vi "Read_Code_Liniarity.vi"(2 "Repeat":i32=1 min=1 max=100, 5 "Port_No":u16=1444, 7 "Core_No":u16=1, 9 "ADC_Controls":T2={"ACQPS"=8, "Break_PT"=0, "Ref_Mod_Sel"=enum."Int_Ref_2P5", "Ref_Sel(Int/Ext)"=enum."Ext", "ADC"=enum."C", "Channel"=15, "LV_samples"=8194, "AGPIO_SEL"=0.0, "LV_perscale"=2, "ODIV"=1, "IMULT"=12}, 11 "error in":errorcluster) -> (4 "max value":u32=4056, 6 "AvgCode":dbl=2038.3436279296875, 8 "min value":u32=20, 15 "error out":errorcluster)   [LabVIEW 2019]
uses:
  Ctrls/ADC_CTRL.ctl
  <userlib>/_TI-LA/Reusable/CCS/APIs/CCS.lvlib
  <userlib>/_TI-LA/Reusable/CCS/APIs/Data/Polymorphics/Read Data From Address - U16 Array.vi
panel:
  in  "Refrence":dbl=2.5 format="%#_13g"
  in  "Sine_Wave_Data_file (use dialog)":path=path "D:/Projects/C2000/Grande/Data/ADC/Group_2/ID_406_AC_Specs/New Text Document.txt"
  out "Tot-Error":u32=4036
  out "Voltage":dbl=1.2441062182188034
  out "ADC_No":u16=2
  out "Waveform Graph":u32[](graph)
  out "Read Data[]":u32[](array[numeric]) format="%#.0f"
  # "1P65-0/2P5-1_Mode_Sel"
  # "LV_Break  = 0;\nUint16 LV_Repeat = 0;\nUint16 LV_Config = 0;\nUint16 LV_samples = 8192;\nUint16 LV_prescale = 2;\nUint16 LV_acqps = 25;\nUint16 LV_AGPIO_TEST = 0;\nUint32 LV_Avg = 0;\nUint16 LV_adcref=   1; // Internal Reference = 0\nUint16 LV_int2p5en= 1; // 2.5V Reference select = 1\nUint16 LV_adcmod =  2; // Adc sel A-0,B-1 & C-2\nUint16 LV_adcchan = 0; // Selecting ADC Channel\nUint16 LV_SYS_MULT =10;"
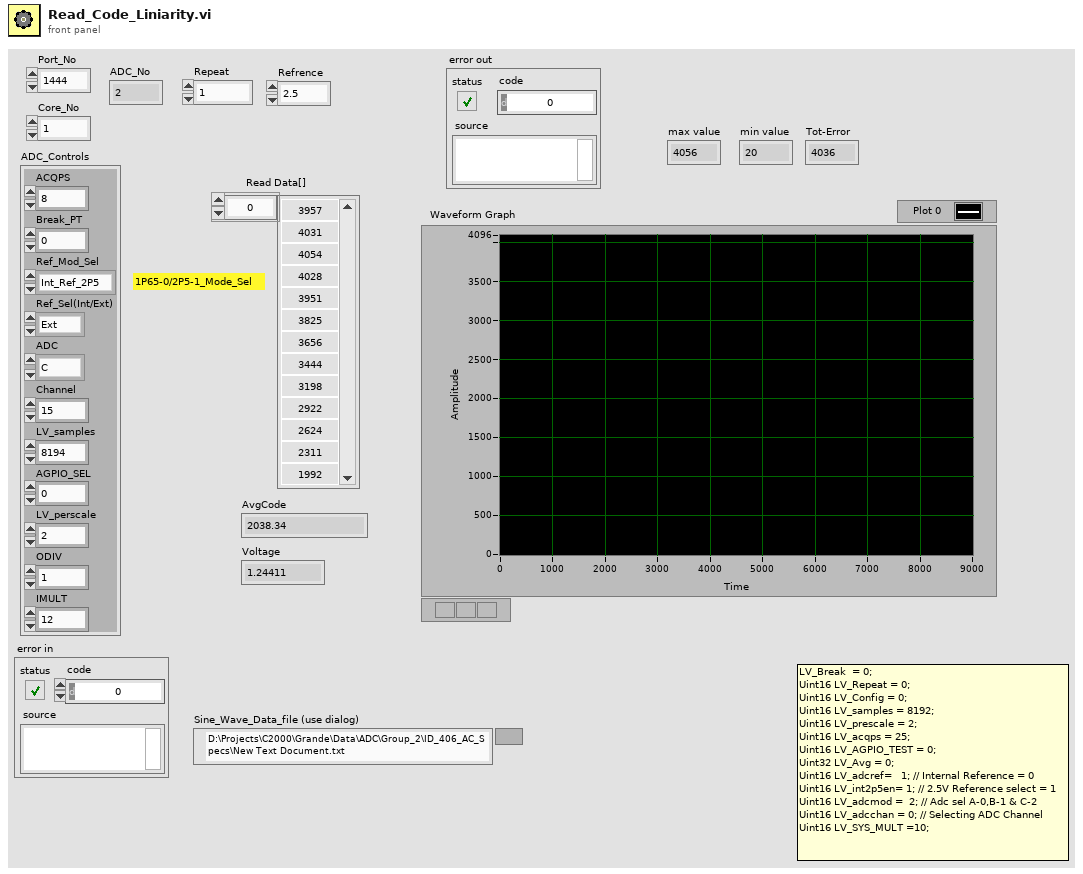
[diagram p1: front panel]
types:
  T1 = typedef "ADC_CTRL.ctl" = enum16{"A", "B", "C"}
  T2 = cluster{"ACQPS":u16, "Break_PT":u16, "Ref_Mod_Sel":enum16{"Int_Ref_1P65", "Int_Ref_2P5"}, "Ref_Sel(Int/Ext)":enum16{"Int", "Ext"}, "ADC":T1, "Channel":u16, "LV_samples":u16, "AGPIO_SEL":dbl, "LV_perscale":u16, "ODIV":u16, "IMULT":u16}
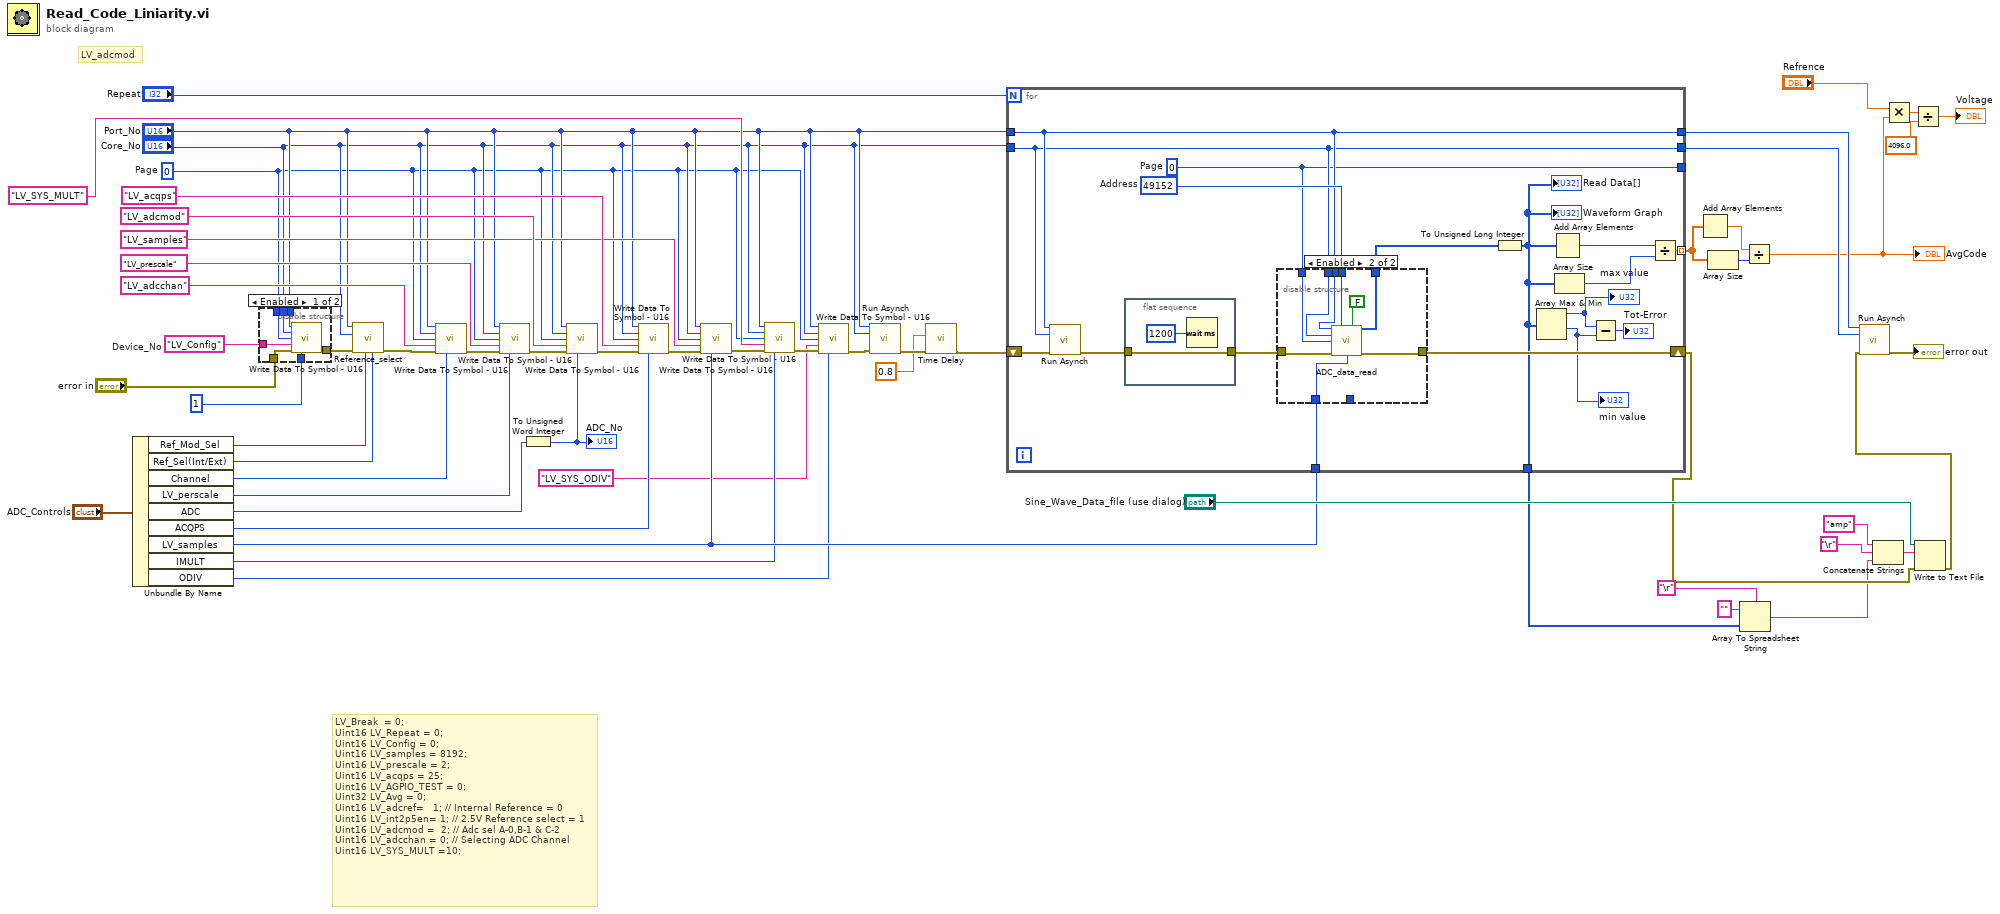
[diagram p0: block diagram]
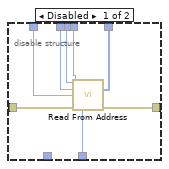
[diagram p3: hidden frame]
diagram:
  w40 = "LV_Config"  # Device_No
  w4 = 0  # Page
  # "LV_Break  = 0;\nUint16 LV_Repeat = 0;\nUint16 LV_Config = 0;\nUint16 LV_samples = 8192;\nUint16 LV_prescale = 2;\nUint16 LV_acqps = 25;\nUint16 LV_AGPIO_TEST = 0;\nUint32 LV_Avg = 0;\nUint16 LV_adcref=   1; // Internal Reference = 0\nUint16 LV_int2p5en= 1; // 2.5V Reference select = 1\nUint16 LV_adcmod =  2; // Adc sel A-0,B-1 & C-2\nUint16 LV_adcchan = 0; // Selecting ADC Channel\nUint16 LV_SYS_MULT =10;"
  # "LV_adcmod"
  n1 = Unbundle By Name("ADC_Controls") -> ("Ref_Mod_Sel"=w31:enum16{"Int_Ref_1P65", "Int_Ref_2P5"}, "Ref_Sel(Int/Ext)"=w30:enum16{"Int", "Ext"}, "Channel"=w29:u16, "LV_perscale"=w28:u16, "ADC"=w27:T1, "ACQPS"=w26:u16, "LV_samples"=w9:u16, "IMULT"=w2:u16, "ODIV"=w3:u16)
  n2 = disable-structure shown="Enabled" {
    disable-tunnel: "error in" -> [w65 _]
    disable-tunnel: w40 -> [w64 _]
    disable-tunnel: w4 -> [w63 _]
    disable-tunnel: [w62 _] -> w39
    disable-tunnel: u16 1 ("Write Data") -> [w61 _]
    disable-tunnel: "Port_No" -> [w60 _]
    disable-tunnel: "Core_No" -> [w59 _]
    frame Enabled {
      n3 = call <userlib>:"Write Data To Symbol - U16.vi"("Port Number"=w60, "Core Number"=w59, "Page"=w63, "Symbol Name"=w64, "error in"=w65, "Write Data"=w61) -> ("error out"=w62:errorcluster)  [unwired: 7 in, 2 out]
    }
    frame Disabled {
    }
  }
  n4 = call "Reference_select.vi"("Ref_Sel(Int/Ext)"=w30, "INT_Ref_Sel"=w31, "error in"=w39, "Core Number"="Core_No", "Port Number"="Port_No") -> ("error out"=w38:errorcluster)  [unwired: 6 in]
  n5 = call <userlib>:"Write Data To Symbol - U16.vi"("Port Number"="Port_No", "Core Number"="Core_No", "Page"=w4, "Symbol Name"="LV_adcchan", "error in"=w38, "Write Data"=w29) -> ("error out"=w57:errorcluster)  [unwired: 7 in, 2 out]
  n6 = call <userlib>:"Write Data To Symbol - U16.vi"("Port Number"="Port_No", "Core Number"="Core_No", "Page"=w4, "Symbol Name"="LV_prescale", "error in"=w57, "Write Data"=w28) -> ("error out"=w56:errorcluster)  [unwired: 7 in, 2 out]
  n7 = To Unsigned Word Integer(number=w27) -> (unsigned 16bit integer=w47:u16)
  "ADC_No" <- w47
  n8 = call <userlib>:"Write Data To Symbol - U16.vi"("Port Number"="Port_No", "Core Number"="Core_No", "Page"=w4, "Symbol Name"="LV_adcmod", "error in"=w56, "Write Data"=w47) -> ("error out"=w58:errorcluster)  [unwired: 7 in, 2 out]
  n9 = call <userlib>:"Write Data To Symbol - U16.vi"("Port Number"="Port_No", "Core Number"="Core_No", "Page"=w4, "Symbol Name"="LV_acqps", "error in"=w58, "Write Data"=w26) -> ("error out"=w51:errorcluster)  [unwired: 7 in, 2 out]
  n10 = call <userlib>:"Write Data To Symbol - U16.vi"("Port Number"="Port_No", "Core Number"="Core_No", "Page"=w4, "Symbol Name"="LV_samples", "error in"=w51, "Write Data"=w9) -> ("error out"=w11:errorcluster)  [unwired: 7 in, 2 out]
  n11 = call <userlib>:"Write Data To Symbol - U16.vi"("Port Number"="Port_No", "Core Number"="Core_No", "Page"=w4, "Symbol Name"="LV_SYS_MULT", "error in"=w11, "Write Data"=w2) -> ("error out"=w8:errorcluster)  [unwired: 7 in, 2 out]
  n12 = call <userlib>:"Write Data To Symbol - U16.vi"("Port Number"="Port_No", "Core Number"="Core_No", "Page"=w4, "Symbol Name"="LV_SYS_ODIV", "error in"=w8, "Write Data"=w3) -> ("error out"=w7:errorcluster)  [unwired: 7 in, 2 out]
  n13 = call <userlib>:"Run Asynch.vi"("Port Number"="Port_No", "Core Number"="Core_No", "error in"=w7) -> ("error out"=w25:errorcluster)  [unwired: 10 in, 2 out]
  n14 = call "Time Delay"("error in (no error)"=w25, "Delay Time (s)"=0.8) -> ("error out"=w24:errorcluster)  [unwired: 9 in]
  n15 = for {
    N: "Repeat" -> [_]
    tunnel: [w79] -> w54 mode=indexing
    tunnel: "Port_No" -> [w75]
    tunnel: "Core_No" -> [w74]
    shift-right: [w78] -> w21
    shift-left: w24 -> [w77]
    tunnel: [w75] -> w50
    tunnel: [w74] -> w49
    tunnel: [w73] -> _
    tunnel: w9 -> [w67]
    tunnel: [w66] -> w13
    w81 = u32 49152  # Address
    w73 = 0  # Page
    n16 = call <userlib>:"Run Asynch.vi"("Port Number"=w75, "Core Number"=w74, "error in"=w77) -> ("error out"=w82:errorcluster)  [unwired: 10 in, 2 out]
    n17 = flat-sequence {
      tunnel: w82 -> [w100]
      tunnel: [w100] -> w72
      frame #0 {
        n18 = Wait (ms)(milliseconds to wait=u32 1200) -> ()  [unwired: 1 out]
      }
    }
    n19 = disable-structure shown="Enabled" {
      disable-tunnel: w81 -> [w90 w95]
      disable-tunnel: [w89 w97] -> w68
      disable-tunnel: [w88 w98] -> w78
      disable-tunnel: w75 -> [w87 w92]
      disable-tunnel: w74 -> [w86 w93]
      disable-tunnel: w73 -> [w85 w94]
      disable-tunnel: w72 -> [w84 w99]
      disable-tunnel: _ -> [w83 _]
      disable-tunnel: w67 -> [_ w96]
      frame Disabled {
        n20 = call-poly <userlib>:"Read From Address.vi"("Port Number"=w87, "Core Number"=w86, "Page"=w85, "Address"=w90, "error in"=w84, "Data Length"=w83) -> ("Read Data[]"=w89:u16[], "error out"=w88:errorcluster)  [unwired: 6 in, 2 out]
      }
      frame Enabled {
        n21 = call "ADC_data_read.vi"("Port Number"=w92, "Address"=w95, "Read_AVG ?"=FALSE, "Core Number"=w93, "Page"=w94, "error in (no error)"=w99, "Lv_Samples"=w96) -> ("Read Data[]"=w97:u16[], "error out"=w98:errorcluster)  [unwired: 6 in, 1 out]
      }
    }
    n22 = To Unsigned Long Integer(number=w68) -> (unsigned 32bit integer=w66:u32[])
    "Waveform Graph" <- w66
    "Read Data[]" <- w66
    n23 = Array Max & Min(array=w66) -> (max value=w71:u32, min value=w70:u32)  [unwired: 2 out]
    "max value" <- w71
    "min value" <- w70
    n24 = Add Array Elements(numeric array=w66) -> (sum=w80:u32)
    n25 = Array Size(array=w66) -> (size(s)=w76:i32)
    n26 = Subtract(x=w71, y=w70) -> (x-y=→"Tot-Error":u32)
    n27 = Divide(x=w80, y=w76) -> (x/y=w79:dbl)
  }
  n28 = Add Array Elements(numeric array=w54) -> (sum=w52:dbl)
  n29 = Array Size(array=w54) -> (size(s)=w53:i32)
  n30 = Array To Spreadsheet String(delimiter (Tab)="\r", array=w13, 3:"" ("format string")) -> (spreadsheet string=w14:string)
  n31 = Divide(x=w52, y=w53) -> (x/y=w46:dbl)
  "AvgCode" <- w46
  n32 = Concatenate Strings("amp", "\r", w14) -> (w18:string)
  n33 = Multiply(x="Refrence", y=w46) -> (x*y=w44:dbl)
  n34 = Divide(x=w44, y=4096.0) -> (x/y=→"Voltage":dbl)
  n35 = Write to Text File(file (use dialog)="Sine_Wave_Data_file (use dialog)", text=w18, error in=w21) -> (error out=w17:errorcluster)  [unwired: 1 in, 2 out]
  n36 = call <userlib>:"Run Asynch.vi"("Port Number"=w50, "Core Number"=w49, "error in"=w17) -> ("error out"=→"error out":errorcluster)  [unwired: 10 in, 2 out]
